vi "Receive All Signals.vi"(8 "error in":errorcluster, 11 "ICAN in":refnum<class "ICAN.lvclass">) -> (0 "error out":errorcluster, 2 "All Signals":T1, 3 "ICAN out":refnum<class "ICAN.lvclass">)   [LabVIEW 2023, in "ICAN.lvclass"]
uses:
  ICAN.lvclass
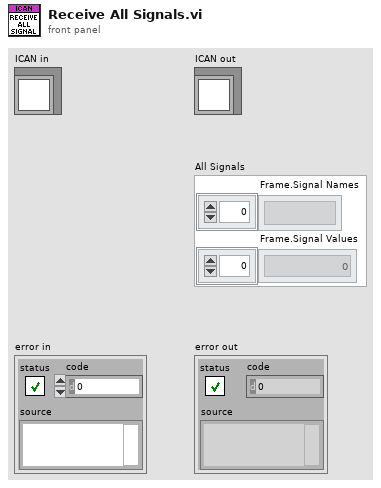
[diagram p1: front panel]
types:
  T1 = cluster{"Frame.Signal Names":string[], "Frame.Signal Values":dbl[]}
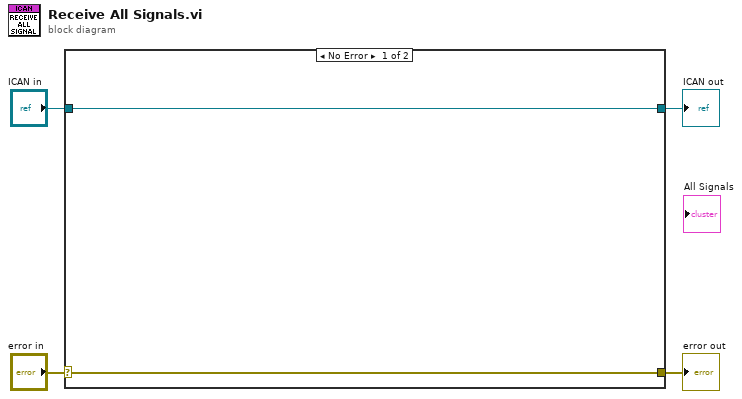
[diagram p0: block diagram]
diagram:
  n1 = case shown="No Error" "error in" {
    selector: "error in" -> [w5 w8]
    tunnel: [w5 w8] -> w3
    tunnel: [w6 w7] -> w1
    tunnel: "ICAN in" -> [w6 w7]
    frame No Error {
    }
    frame Error {
    }
  }
  "error out" <- w3
  "ICAN out" <- w1
